vi "vr-main-window.vi"(10 "Robot Num":enum16{"Rob-One", "Rob-Two"}(ring), 11 "EventIn":refnum<class "NISAST Event.lvclass">) -> ()   [LabVIEW 2013]
uses:
  <resource>/importtools/Common/Event/NISAST Event.lvclass
  vr-states.ctl
  <vilib>/picture/3D Picture Control/NI_3D Picture Control.lvlib
panel:
  in  "StopFour":bool
  in  "ClockWise":bool
  in  "AntiClockWise":bool
  in  "Up":bool
  in  "Down":bool
  out "Event Message":string
  out "StopVRWindow?":bool
  in  "Stop":bool
  # "这个名字千万不能改"
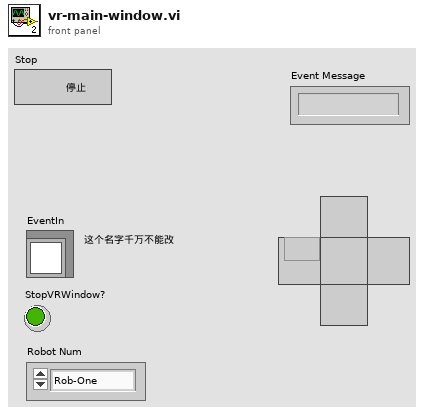
[diagram p1: front panel]
types:
  T1 = typedef "vr-states.ctl" = enum16{"init", "wait", "stopVR", "Ro-Up", "Ro-Down", "Ro-Clockwise", "Ro-AntiClock", "Ro-Stop"}
  T2 = enum16{"Open", "Minimized", "Maximized", "Hidden"}
  T3 = cluster{"zuoqian1":refnum<vi>, "zuoqian2":refnum<vi>, "zuoqian3":refnum<vi>}
  T4 = cluster{"zuohou1":refnum<vi>, "zuohou2":refnum<vi>, "zuohou3":refnum<vi>}
  T5 = cluster{"youqian1":refnum<vi>, "youqian2":refnum<vi>, "youqian3":refnum<vi>}
  T6 = cluster{"youhou1":refnum<vi>, "youhou2":refnum<vi>, "youhou3":refnum<vi>}
  T7 = enum16{"None", "Spherical", "Flying", "Oriented"}
  T8 = typedef "NISAST Event.lvclass/Event Registeration Refnum.ctl" = refnum<event-registration>
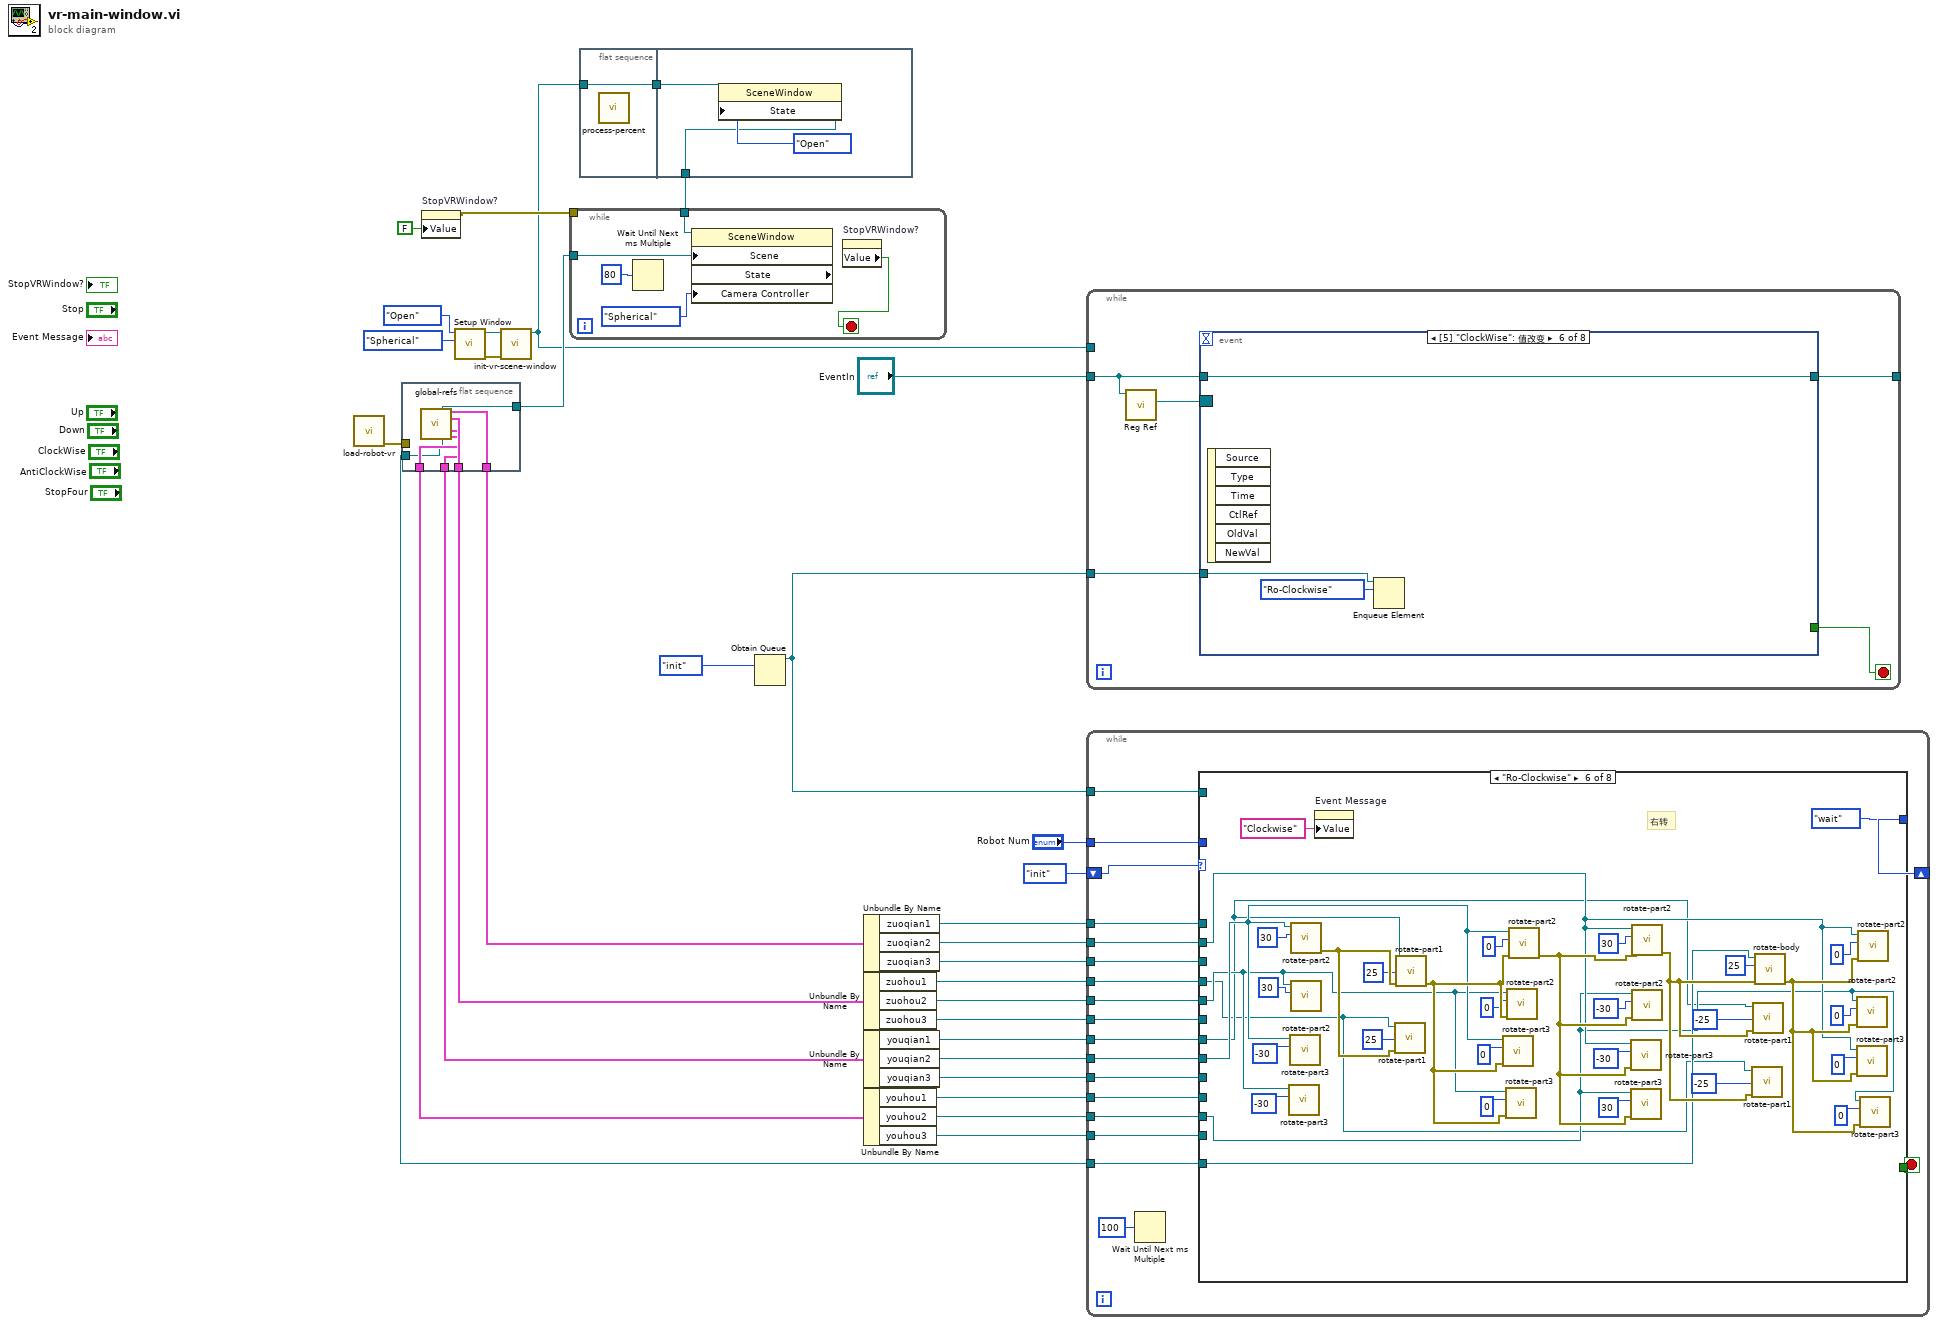
[diagram p0: block diagram]
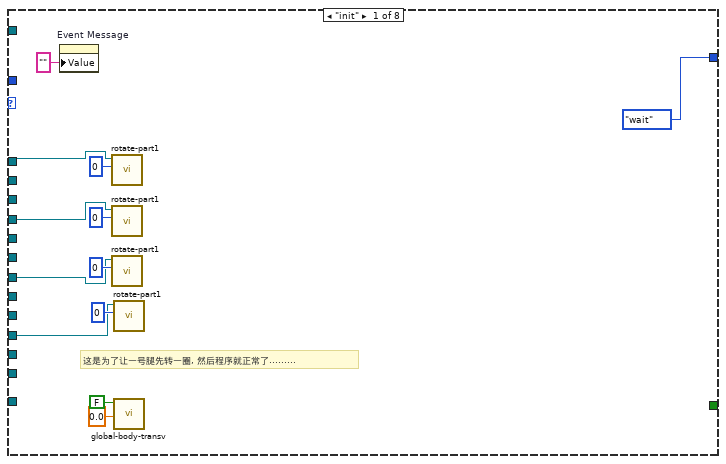
[diagram p2: hidden frame]
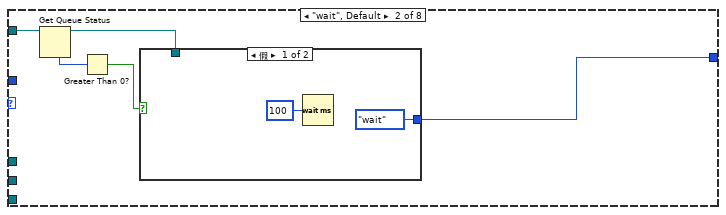
[diagram p3: hidden frame]
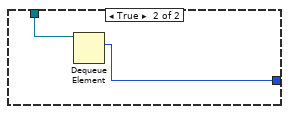
[diagram p4: hidden frame]
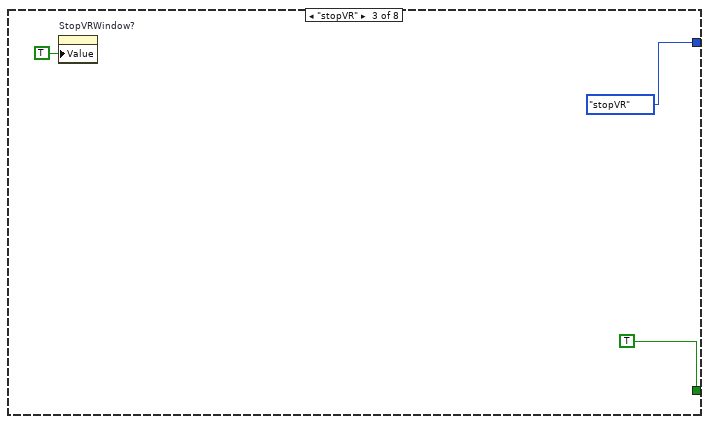
[diagram p5: hidden frame]
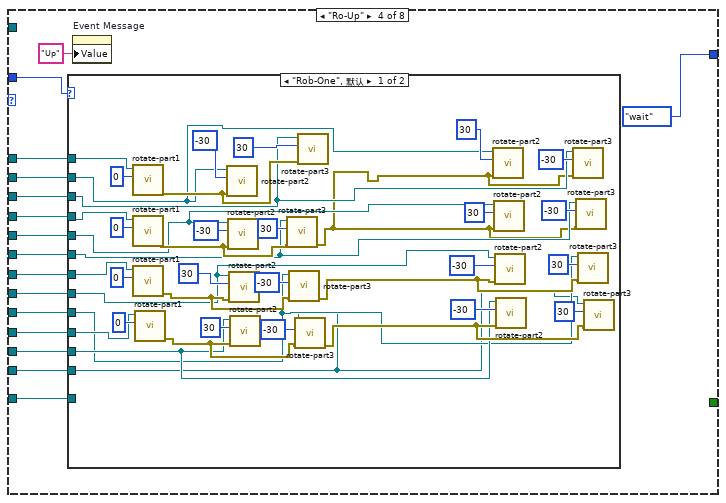
[diagram p6: hidden frame]
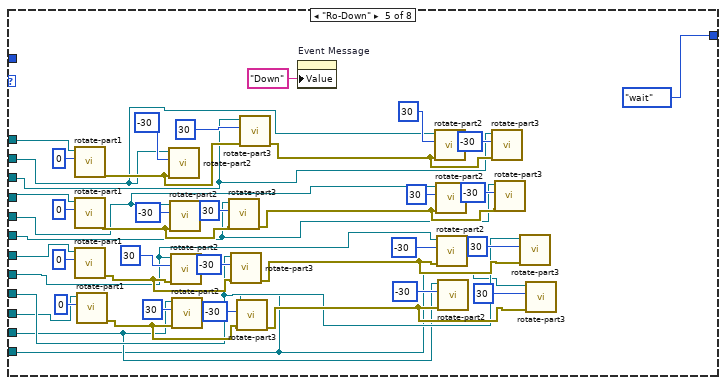
[diagram p8: hidden frame]
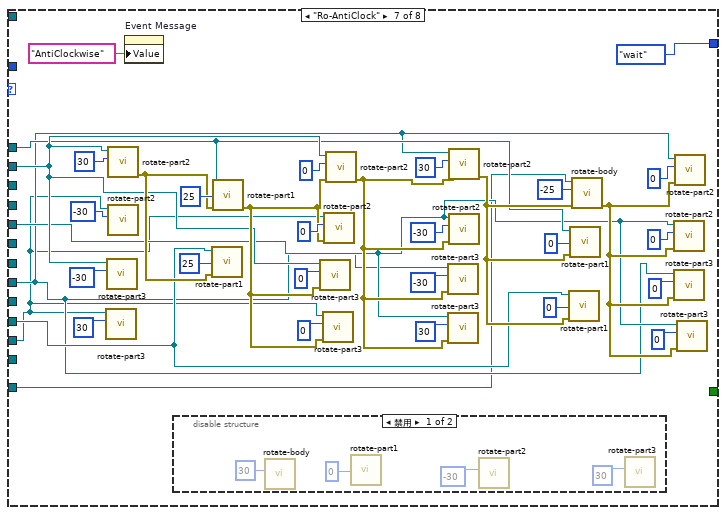
[diagram p9: hidden frame]
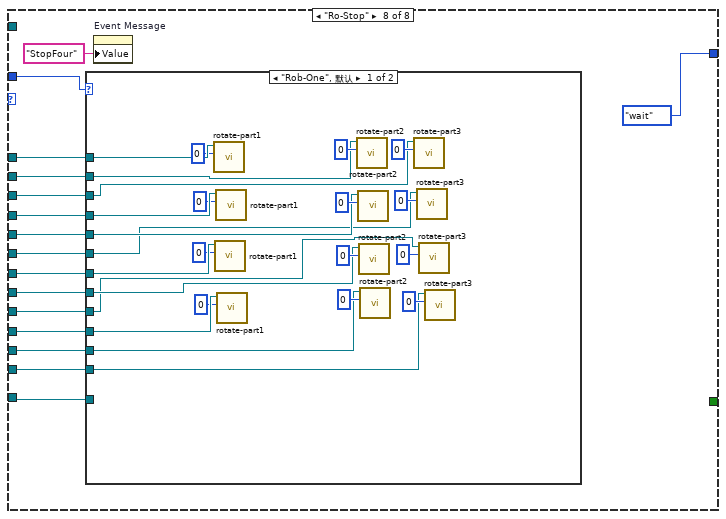
[diagram p11: hidden frame]
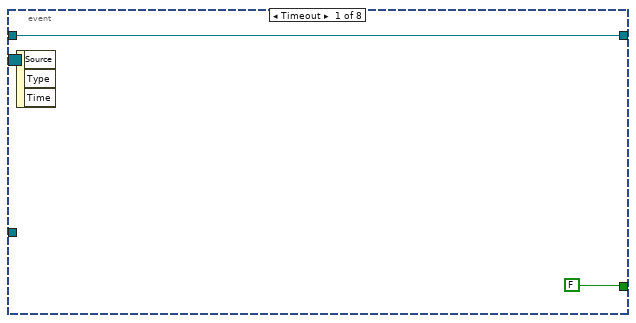
[diagram p13: hidden frame]
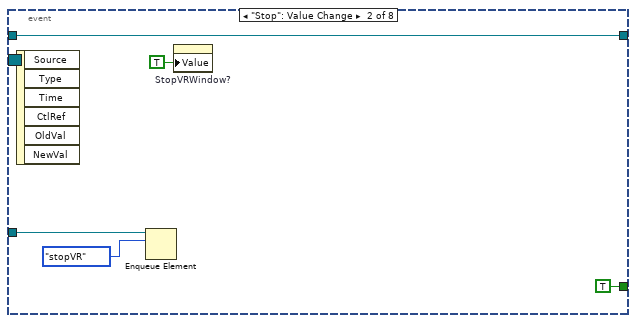
[diagram p14: hidden frame]
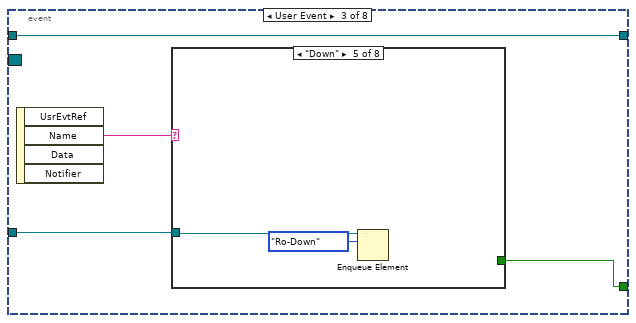
[diagram p15: hidden frame]
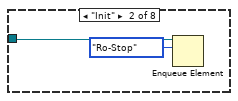
[diagram p17: hidden frame]
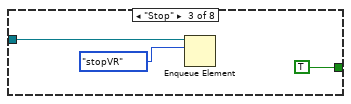
[diagram p18: hidden frame]
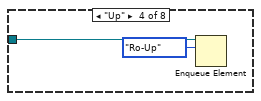
[diagram p19: hidden frame]
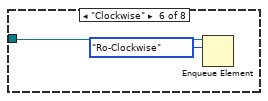
[diagram p20: hidden frame]
diagram:
  n1 = call "load-robot-vr.vi"() -> ("错误输出"=w29:errorcluster)  [unwired: 11 in]
  n2 = flat-sequence {
    tunnel: [w39] -> w27
    tunnel: w29 -> [_]
    tunnel: [w38] -> w28
    tunnel: [w37] -> w21
    tunnel: [w36] -> w20
    tunnel: [w35] -> w19
    tunnel: [w34] -> w6
    frame #0 {
      n3 = call "global-refs.vi"() -> ("RobotRef"=w39:refnum<vi>, "ZuoQianRef"=w38:T3, "ZuoHouRef"=w37:T4, "YouQianRef"=w36:T5, "BodyRef"=w34:refnum<vi>, "YouHouRef"=w35:T6)  [unwired: 10 in]
    }
  }
  n4 = property on="StopVRWindow?" class="Bool (严格)"("Value"=FALSE ("StopVRWindow?")) -> (error out=w4:errorcluster)  [unwired: 2 in, 1 out]
  n5 = call <vilib>:"Setup Window.vi"("Camera Controller"=enum16{"None", "Spherical", "Flying"}."Spherical", "Window State"=T2."Open") -> ("error out"=w33:errorcluster, "New Window Refnum"=w32:refnum<vi>)  [unwired: 1 in, 7 out]
  n6 = call "init-vr-scene-window.vi"("错误输入（无错误）"=w33, "SceneWindow输入"=w32) -> ("SceneWindow输出"=w3:refnum<vi>)  [unwired: 8 in, 1 out]
  n7 = while {
    tunnel: w27 -> [w43]
    tunnel: w1 -> [w42]
    tunnel: w4 -> [_]
    stop <- w40 stop-if-true
    n8 = Wait Until Next ms Multiple(millisecond multiple=u32 80 ("毫秒倍数")) -> ()  [unwired: 1 out]
    n9 = property class="SceneWindow" props=["Scene", "State", "Camera Controller"](reference=w42, "Scene"=w43, "Camera Controller"=T7."Spherical" ("视角控制器:类型")) -> ()  [unwired: 1 in, 3 out]
    n10 = property on="StopVRWindow?" class="Bool (严格)"() -> ("Value"=w40:bool)  [unwired: 2 in, 2 out]
  }
  n11 = flat-sequence {
    tunnel: w3 -> [w45]
    tunnel: [w45] -> w2
    tunnel: w2 -> [w47]
    tunnel: [w46] -> w1
    frame #0 {
      n12 = call "process-percent.vi"() -> ()  [unwired: 12 in]
    }
    frame #1 {
      n13 = property class="SceneWindow"(reference=w47, "State"=T2."Open" ("窗口状态")) -> (reference out=w46:refnum<vi>)  [unwired: 1 in, 1 out]
    }
  }
  n14 = Obtain Queue(element data type=vr-states."init" ("States")) -> (queue out=w25:refnum<queue>)  [unwired: 4 in, 2 out]
  n15 = Unbundle By Name(w28) -> ("zuoqian1"=w18:refnum<vi>, "zuoqian2"=w17:refnum<vi>, "zuoqian3"=w16:refnum<vi>)
  n16 = Unbundle By Name(w21) -> ("zuohou1"=w15:refnum<vi>, "zuohou2"=w14:refnum<vi>, "zuohou3"=w13:refnum<vi>)
  n17 = Unbundle By Name(w20) -> ("youqian1"=w12:refnum<vi>, "youqian2"=w11:refnum<vi>, "youqian3"=w10:refnum<vi>)
  n18 = Unbundle By Name(w19) -> ("youhou1"=w9:refnum<vi>, "youhou2"=w8:refnum<vi>, "youhou3"=w7:refnum<vi>)
  n19 = while {
    tunnel: w3 -> [_]
    tunnel: w25 -> [w53]
    tunnel: "EventIn" -> [w51]
    tunnel: [w49] -> _
    stop <- w52 stop-if-true
    n20 = call-dynamic "Reg Ref.vi"("Event in"=w51) -> ("Event Registration Refnum"=w50:T8)  [unwired: 8 in, 2 out]
    n21 = event shown="[5] \"ClockWise\": 值改变" {
      selector: w50 -> [_ _ _ _ _ _ _ _]
      dyn-events: _ -> [_ _ _ _ _ _ _ _]
      timeout: _ -> [_ _ _ _ _ _ _ _]
      tunnel: w53 -> [_ w59 w63 w81 w84 w87 w90 w93]
      tunnel: [FALSE TRUE w62 _ _ _ _ _] -> w52
      tunnel: w51 -> [w54 w56 w61 w80 w83 w86 w89 w92]
      tunnel: [w54 w56 w61 w80 w83 w86 w89 w92] -> w49
      event Timeout {
        n22 = event-data() -> ()  [unwired: 1 in, 3 out]
      }
      event "Stop": Value Change {
        n23 = event-data() -> ()  [unwired: 1 in, 6 out]
        n24 = Enqueue Element(queue=w59, element=vr-states."stopVR" ("元素")) -> ()  [unwired: 2 in, 3 out]
        n25 = property on="StopVRWindow?" class="Bool (严格)"("Value"=TRUE ("StopVRWindow?")) -> ()  [unwired: 2 in, 2 out]
      }
      event User Event {
        n26 = event-data() -> ("Name"=w64:string)  [unwired: 1 in, 3 out]
        n27 = case shown="\"Down\"" w64 {
          tunnel: w63 -> [_ w66 w68 w70 w72 w74 w76 w78]
          tunnel: [_ _ TRUE _ _ _ _ _] -> w62
          frame "none", Default {
          }
          frame "Init" {
            n28 = Enqueue Element(queue=w66, element=vr-states."Ro-Stop" ("元素")) -> ()  [unwired: 2 in, 3 out]
          }
          frame "Stop" {
            n29 = Enqueue Element(queue=w68, element=vr-states."stopVR" ("元素")) -> ()  [unwired: 2 in, 3 out]
          }
          frame "Up" {
            n30 = Enqueue Element(queue=w70, element=vr-states."Ro-Up" ("元素")) -> ()  [unwired: 2 in, 3 out]
          }
          frame "Down" {
            n31 = Enqueue Element(queue=w72, element=vr-states."Ro-Down" ("元素")) -> ()  [unwired: 2 in, 3 out]
          }
          frame "Clockwise" {
            n32 = Enqueue Element(queue=w74, element=vr-states."Ro-Clockwise" ("元素")) -> ()  [unwired: 2 in, 3 out]
          }
          frame "AntiClockwise" {
            n33 = Enqueue Element(queue=w76, element=vr-states."Ro-AntiClock" ("元素")) -> ()  [unwired: 2 in, 3 out]
          }
          frame "StopFour" {
            n34 = Enqueue Element(queue=w78, element=vr-states."Ro-Stop" ("元素")) -> ()  [unwired: 2 in, 3 out]
          }
        }
      }
      event "Up": Value Change {
        n35 = event-data() -> ()  [unwired: 1 in, 6 out]
        n36 = Enqueue Element(queue=w81, element=vr-states."Ro-Up" ("元素")) -> ()  [unwired: 2 in, 3 out]
      }
      event "Down": Value Change {
        n37 = event-data() -> ()  [unwired: 1 in, 6 out]
        n38 = Enqueue Element(queue=w84, element=vr-states."Ro-Down" ("元素")) -> ()  [unwired: 2 in, 3 out]
      }
      event "ClockWise": Value Change {
        n39 = event-data() -> ()  [unwired: 1 in, 6 out]
        n40 = Enqueue Element(queue=w87, element=vr-states."Ro-Clockwise" ("元素")) -> ()  [unwired: 2 in, 3 out]
      }
      event "AntiClockWise": Value Change {
        n41 = event-data() -> ()  [unwired: 1 in, 6 out]
        n42 = Enqueue Element(queue=w90, element=vr-states."Ro-AntiClock" ("元素")) -> ()  [unwired: 2 in, 3 out]
      }
      event "StopFour": Value Change {
        n43 = event-data() -> ()  [unwired: 1 in, 6 out]
        n44 = Enqueue Element(queue=w93, element=vr-states."Ro-Stop" ("元素")) -> ()  [unwired: 2 in, 3 out]
      }
    }
  }
  n45 = while {
    tunnel: w25 -> [w112]
    shift-right: [w111] -> _
    shift-left: vr-states."init" ("States") -> [w110]
    tunnel: "Robot Num" -> [w109]
    tunnel: w18 -> [w108]
    tunnel: w17 -> [w107]
    tunnel: w16 -> [w106]
    tunnel: w15 -> [w105]
    tunnel: w14 -> [w104]
    tunnel: w13 -> [w103]
    tunnel: w12 -> [w102]
    tunnel: w11 -> [w101]
    tunnel: w10 -> [w100]
    tunnel: w9 -> [w99]
    tunnel: w8 -> [w98]
    tunnel: w7 -> [w97]
    tunnel: w6 -> [w95]
    stop <- w113 stop-if-true
    n46 = Wait Until Next ms Multiple(millisecond multiple=u32 100 ("毫秒倍数")) -> ()  [unwired: 1 out]
    n47 = case shown="\"Ro-Clockwise\"" w110 {
      tunnel: [_ _ TRUE _ _ _ _ _] -> w113
      tunnel: w112 -> [_ w130 _ _ _ _ _ _]
      tunnel: [vr-states."wait" ("States") w126 vr-states."stopVR" ("States") vr-states."wait" ("States") vr-states."wait" ("States") vr-states."wait" ("States") vr-states."wait" ("States") vr-states."wait" ("States")] -> w111
      tunnel: w109 -> [_ _ _ w148 _ _ _ w322]
      tunnel: w108 -> [w119 _ _ w151 w204 _ w275 w321]
      tunnel: w107 -> [_ _ _ w150 w203 w259 w276 w320]
      tunnel: w106 -> [_ _ _ w149 w202 _ _ w319]
      tunnel: w105 -> [w118 _ _ w147 w201 w256 _ w318]
      tunnel: w104 -> [_ _ _ w146 w200 w261 w274 w317]
      tunnel: w103 -> [_ _ _ w145 w199 _ _ w316]
      tunnel: w102 -> [w117 _ _ w144 w198 w257 _ w315]
      tunnel: w101 -> [_ _ _ w143 w197 w262 w272 w314]
      tunnel: w100 -> [_ _ _ w142 w196 _ _ w313]
      tunnel: w99 -> [w116 _ _ w141 w195 _ w273 w312]
      tunnel: w98 -> [_ _ _ w140 w194 w258 w271 w311]
      tunnel: w97 -> [_ _ _ w139 w193 _ _ w310]
      tunnel: w95 -> [_ _ _ w138 _ w260 w270 w309]
      frame "init" {
        # "这是为了让一号腿先转一圈, 然后程序就正常了........."
        n48 = property on="Event Message" class="Str"("Value"="" ("Event Message")) -> ()  [unwired: 2 in, 2 out]
        n49 = call "rotate-part1.vi"("Angle"=0, "SceneObject输入"=w119) -> ()  [unwired: 8 in, 2 out]
        n50 = call "rotate-part1.vi"("Angle"=0, "SceneObject输入"=w118) -> ()  [unwired: 8 in, 2 out]
        n51 = call "rotate-part1.vi"("Angle"=0, "SceneObject输入"=w117) -> ()  [unwired: 8 in, 2 out]
        n52 = call "rotate-part1.vi"("Angle"=0, "SceneObject输入"=w116) -> ()  [unwired: 8 in, 2 out]
        n53 = call "global-body-transv.vi"("rad"=0.0, "Read?"=FALSE) -> ()  [unwired: 8 in, 2 out]
      }
      frame "wait", Default {
        n54 = Get Queue Status(queue=w130) -> (queue out=w127:refnum<queue>, # elements in queue=w129:i32)  [unwired: 2 in, 6 out]
        n55 = Greater Than 0?(x=w129) -> (x > 0?=w128:bool)
        n56 = case shown="假" w128 {
          tunnel: w127 -> [_ w134]
          tunnel: [vr-states."wait" ("States") w133] -> w126
          frame False {
            n57 = Wait (ms)(milliseconds to wait=u32 100 ("等待时间（毫秒）")) -> ()  [unwired: 1 out]
          }
          frame True {
            n58 = Dequeue Element(queue=w134) -> (element=w133:T1)  [unwired: 2 in, 3 out]
          }
        }
      }
      frame "stopVR" {
        n59 = property on="StopVRWindow?" class="Bool (严格)"("Value"=TRUE ("StopVRWindow?")) -> ()  [unwired: 2 in, 2 out]
      }
      frame "Ro-Up" {
        n60 = case shown="\"Rob-One\", 默认" w148 {
          tunnel: w151 -> [w188 _]
          tunnel: w150 -> [w162 _]
          tunnel: w149 -> [w159 _]
          tunnel: w147 -> [w187 _]
          tunnel: w146 -> [w161 _]
          tunnel: w145 -> [w158 _]
          tunnel: w144 -> [w186 _]
          tunnel: w143 -> [w157 _]
          tunnel: w142 -> [w156 _]
          tunnel: w141 -> [w185 _]
          tunnel: w140 -> [w160 _]
          tunnel: w139 -> [w155 _]
          tunnel: w138 -> [_ _]
          frame "Rob-One", Default {
            n61 = call "rotate-part1.vi"("Angle"=0, "SceneObject输入"=w188) -> ("Error Out"=w180:errorcluster)  [unwired: 8 in, 1 out]
            n62 = call "rotate-part1.vi"("Angle"=0, "SceneObject输入"=w187) -> ("Error Out"=w179:errorcluster)  [unwired: 8 in, 1 out]
            n63 = call "rotate-part1.vi"("Angle"=0, "SceneObject输入"=w186) -> ("Error Out"=w178:errorcluster)  [unwired: 8 in, 1 out]
            n64 = call "rotate-part1.vi"("Angle"=0, "SceneObject输入"=w185) -> ("Error Out"=w177:errorcluster)  [unwired: 8 in, 1 out]
            n65 = call "rotate-part2.vi"("Error In"=w180, "Angle"=-30, "SceneObject输入"=w162) -> ()  [unwired: 7 in, 2 out]
            n66 = call "rotate-part2.vi"("Error In"=w179, "Angle"=-30, "SceneObject输入"=w161) -> ()  [unwired: 7 in, 2 out]
            n67 = call "rotate-part2.vi"("Error In"=w178, "Angle"=30, "SceneObject输入"=w157) -> ()  [unwired: 7 in, 2 out]
            n68 = call "rotate-part2.vi"("Error In"=w177, "Angle"=30, "SceneObject输入"=w160) -> ()  [unwired: 7 in, 2 out]
            n69 = call "rotate-part3.vi"("Error In"=w179, "Angle"=30, "SceneObject输入"=w158) -> ("Error Out"=w154:errorcluster)  [unwired: 7 in, 1 out]
            n70 = call "rotate-part3.vi"("Error In"=w178, "Angle"=-30, "SceneObject输入"=w156) -> ("Error Out"=w164:errorcluster)  [unwired: 7 in, 1 out]
            n71 = call "rotate-part3.vi"("Error In"=w177, "Angle"=-30, "SceneObject输入"=w155) -> ("Error Out"=w163:errorcluster)  [unwired: 7 in, 1 out]
            n72 = call "rotate-part3.vi"("Error In"=w180, "Angle"=30, "SceneObject输入"=w159) -> ()  [unwired: 7 in, 2 out]
            n73 = call "rotate-part2.vi"("Error In"=w154, "Angle"=30, "SceneObject输入"=w162) -> ()  [unwired: 7 in, 2 out]
            n74 = call "rotate-part2.vi"("Error In"=w154, "Angle"=30, "SceneObject输入"=w161) -> ()  [unwired: 7 in, 2 out]
            n75 = call "rotate-part2.vi"("Error In"=w164, "Angle"=-30, "SceneObject输入"=w157) -> ()  [unwired: 7 in, 2 out]
            n76 = call "rotate-part2.vi"("Error In"=w163, "Angle"=-30, "SceneObject输入"=w160) -> ()  [unwired: 7 in, 2 out]
            n77 = call "rotate-part3.vi"("Error In"=w154, "Angle"=-30, "SceneObject输入"=w159) -> ()  [unwired: 7 in, 2 out]
            n78 = call "rotate-part3.vi"("Error In"=w154, "Angle"=-30, "SceneObject输入"=w158) -> ()  [unwired: 7 in, 2 out]
            n79 = call "rotate-part3.vi"("Error In"=w164, "Angle"=30, "SceneObject输入"=w156) -> ()  [unwired: 7 in, 2 out]
            n80 = call "rotate-part3.vi"("Error In"=w163, "Angle"=30, "SceneObject输入"=w155) -> ()  [unwired: 7 in, 2 out]
          }
          frame "Rob-Two" {
          }
        }
        n81 = property on="Event Message" class="Str"("Value"="Up" ("Event Message")) -> ()  [unwired: 2 in, 2 out]
      }
      frame "Ro-Down" {
        n82 = call "rotate-part1.vi"("Angle"=0, "SceneObject输入"=w204) -> ("Error Out"=w224:errorcluster)  [unwired: 8 in, 1 out]
        n83 = call "rotate-part1.vi"("Angle"=0, "SceneObject输入"=w201) -> ("Error Out"=w223:errorcluster)  [unwired: 8 in, 1 out]
        n84 = call "rotate-part1.vi"("Angle"=0, "SceneObject输入"=w198) -> ("Error Out"=w222:errorcluster)  [unwired: 8 in, 1 out]
        n85 = call "rotate-part1.vi"("Angle"=0, "SceneObject输入"=w195) -> ("Error Out"=w221:errorcluster)  [unwired: 8 in, 1 out]
        n86 = call "rotate-part2.vi"("Error In"=w224, "Angle"=-30, "SceneObject输入"=w203) -> ()  [unwired: 7 in, 2 out]
        n87 = call "rotate-part2.vi"("Error In"=w223, "Angle"=-30, "SceneObject输入"=w200) -> ()  [unwired: 7 in, 2 out]
        n88 = call "rotate-part2.vi"("Error In"=w222, "Angle"=30, "SceneObject输入"=w197) -> ()  [unwired: 7 in, 2 out]
        n89 = call "rotate-part2.vi"("Error In"=w221, "Angle"=30, "SceneObject输入"=w194) -> ()  [unwired: 7 in, 2 out]
        n90 = call "rotate-part3.vi"("Error In"=w223, "Angle"=30, "SceneObject输入"=w199) -> ("Error Out"=w207:errorcluster)  [unwired: 7 in, 1 out]
        n91 = call "rotate-part3.vi"("Error In"=w222, "Angle"=-30, "SceneObject输入"=w196) -> ("Error Out"=w206:errorcluster)  [unwired: 7 in, 1 out]
        n92 = call "rotate-part3.vi"("Error In"=w221, "Angle"=-30, "SceneObject输入"=w193) -> ("Error Out"=w205:errorcluster)  [unwired: 7 in, 1 out]
        n93 = call "rotate-part3.vi"("Error In"=w224, "Angle"=30, "SceneObject输入"=w202) -> ("Error Out"=w208:errorcluster)  [unwired: 7 in, 1 out]
        n94 = property on="Event Message" class="Str"("Value"="Down" ("Event Message")) -> ()  [unwired: 2 in, 2 out]
        n95 = call "rotate-part2.vi"("Error In"=w208, "Angle"=30, "SceneObject输入"=w203) -> ()  [unwired: 7 in, 2 out]
        n96 = call "rotate-part2.vi"("Error In"=w207, "Angle"=30, "SceneObject输入"=w200) -> ()  [unwired: 7 in, 2 out]
        n97 = call "rotate-part2.vi"("Error In"=w206, "Angle"=-30, "SceneObject输入"=w197) -> ()  [unwired: 7 in, 2 out]
        n98 = call "rotate-part2.vi"("Error In"=w205, "Angle"=-30, "SceneObject输入"=w194) -> ()  [unwired: 7 in, 2 out]
        n99 = call "rotate-part3.vi"("Error In"=w208, "Angle"=-30, "SceneObject输入"=w202) -> ()  [unwired: 7 in, 2 out]
        n100 = call "rotate-part3.vi"("Error In"=w207, "Angle"=-30, "SceneObject输入"=w199) -> ()  [unwired: 7 in, 2 out]
        n101 = call "rotate-part3.vi"("Error In"=w206, "Angle"=30, "SceneObject输入"=w196) -> ()  [unwired: 7 in, 2 out]
        n102 = call "rotate-part3.vi"("Error In"=w205, "Angle"=30, "SceneObject输入"=w193) -> ()  [unwired: 7 in, 2 out]
      }
      frame "Ro-Clockwise" {
        # "右转"
        n103 = call "rotate-part3.vi"("Angle"=-30, "SceneObject输入"=w261) -> ()  [unwired: 8 in, 2 out]
        n104 = call "rotate-part3.vi"("Angle"=-30, "SceneObject输入"=w262) -> ()  [unwired: 8 in, 2 out]
        n105 = call "rotate-part2.vi"("Angle"=30, "SceneObject输入"=w262) -> ("Error Out"=w267:errorcluster)  [unwired: 8 in, 1 out]
        n106 = call "rotate-part2.vi"("Angle"=30, "SceneObject输入"=w261) -> ()  [unwired: 8 in, 2 out]
        n107 = property on="Event Message" class="Str"("Value"="Clockwise" ("Event Message")) -> ()  [unwired: 2 in, 2 out]
        n108 = call "rotate-part1.vi"("Error In"=w267, "Angle"=25, "SceneObject输入"=w256) -> ()  [unwired: 7 in, 2 out]
        n109 = call "rotate-part1.vi"("Error In"=w267, "Angle"=25, "SceneObject输入"=w257) -> ("Error Out"=w265:errorcluster)  [unwired: 7 in, 1 out]
        n110 = call "rotate-part3.vi"("Error In"=w265, "Angle"=0, "SceneObject输入"=w262) -> ()  [unwired: 7 in, 2 out]
        n111 = call "rotate-part3.vi"("Error In"=w265, "Angle"=0, "SceneObject输入"=w261) -> ()  [unwired: 7 in, 2 out]
        n112 = call "rotate-part2.vi"("Error In"=w265, "Angle"=0, "SceneObject输入"=w261) -> ()  [unwired: 7 in, 2 out]
        n113 = call "rotate-part2.vi"("Error In"=w265, "Angle"=0, "SceneObject输入"=w262) -> ("Error Out"=w266:errorcluster)  [unwired: 7 in, 1 out]
        n114 = call "rotate-part3.vi"("Error In"=w266, "Angle"=-30, "SceneObject输入"=w259) -> ()  [unwired: 7 in, 2 out]
        n115 = call "rotate-part3.vi"("Error In"=w266, "Angle"=30, "SceneObject输入"=w258) -> ()  [unwired: 7 in, 2 out]
        n116 = call "rotate-part2.vi"("Error In"=w266, "Angle"=30, "SceneObject输入"=w259) -> ("Error Out"=w264:errorcluster)  [unwired: 7 in, 1 out]
        n117 = call "rotate-part2.vi"("Error In"=w266, "Angle"=-30, "SceneObject输入"=w258) -> ()  [unwired: 7 in, 2 out]
        n118 = call "rotate-part1.vi"("Error In"=w264, "Angle"=-25, "SceneObject输入"=w256) -> ()  [unwired: 7 in, 2 out]
        n119 = call "rotate-part1.vi"("Error In"=w264, "Angle"=-25, "SceneObject输入"=w257) -> ()  [unwired: 7 in, 2 out]
        n120 = call "rotate-body.vi"("Error In"=w264, "Angle"=25, "SceneObject输入"=w260) -> ("Error Out"=w263:errorcluster)  [unwired: 7 in, 1 out]
        n121 = call "rotate-part2.vi"("Error In"=w263, "Angle"=0, "SceneObject输入"=w258) -> ()  [unwired: 7 in, 2 out]
        n122 = call "rotate-part3.vi"("Error In"=w263, "Angle"=0, "SceneObject输入"=w259) -> ()  [unwired: 7 in, 2 out]
        n123 = call "rotate-part2.vi"("Error In"=w263, "Angle"=0, "SceneObject输入"=w259) -> ()  [unwired: 7 in, 2 out]
        n124 = call "rotate-part3.vi"("Error In"=w263, "Angle"=0, "SceneObject输入"=w258) -> ()  [unwired: 7 in, 2 out]
      }
      frame "Ro-AntiClock" {
        n125 = call "rotate-part3.vi"("Angle"=30, "SceneObject输入"=w271) -> ()  [unwired: 8 in, 2 out]
        n126 = call "rotate-part3.vi"("Angle"=-30, "SceneObject输入"=w276) -> ()  [unwired: 8 in, 2 out]
        n127 = call "rotate-part2.vi"("Angle"=30, "SceneObject输入"=w276) -> ("Error Out"=w282:errorcluster)  [unwired: 8 in, 1 out]
        n128 = call "rotate-part2.vi"("Angle"=-30, "SceneObject输入"=w271) -> ()  [unwired: 8 in, 2 out]
        n129 = property on="Event Message" class="Str"("Value"="AntiClockwise" ("Event Message")) -> ()  [unwired: 2 in, 2 out]
        n130 = disable-structure shown="禁用" {
          frame Disabled {
            n131 = call "rotate-body.vi"("Angle"=30) -> ()  [unwired: 9 in, 2 out]
            n132 = call "rotate-part1.vi"("Angle"=0) -> ()  [unwired: 9 in, 2 out]
            n133 = call "rotate-part2.vi"("Angle"=-30) -> ()  [unwired: 9 in, 2 out]
            n134 = call "rotate-part3.vi"("Angle"=30) -> ()  [unwired: 9 in, 2 out]
          }
          frame Enabled {
          }
        }
        n135 = call "rotate-part1.vi"("Error In"=w282, "Angle"=25, "SceneObject输入"=w273) -> ()  [unwired: 7 in, 2 out]
        n136 = call "rotate-part1.vi"("Error In"=w282, "Angle"=25, "SceneObject输入"=w275) -> ("Error Out"=w280:errorcluster)  [unwired: 7 in, 1 out]
        n137 = call "rotate-part3.vi"("Error In"=w280, "Angle"=0, "SceneObject输入"=w276) -> ()  [unwired: 7 in, 2 out]
        n138 = call "rotate-part3.vi"("Error In"=w280, "Angle"=0, "SceneObject输入"=w271) -> ()  [unwired: 7 in, 2 out]
        n139 = call "rotate-part2.vi"("Error In"=w280, "Angle"=0, "SceneObject输入"=w271) -> ()  [unwired: 7 in, 2 out]
        n140 = call "rotate-part2.vi"("Error In"=w280, "Angle"=0, "SceneObject输入"=w276) -> ("Error Out"=w281:errorcluster)  [unwired: 7 in, 1 out]
        n141 = call "rotate-part3.vi"("Error In"=w281, "Angle"=-30, "SceneObject输入"=w272) -> ()  [unwired: 7 in, 2 out]
        n142 = call "rotate-part3.vi"("Error In"=w281, "Angle"=30, "SceneObject输入"=w274) -> ()  [unwired: 7 in, 2 out]
        n143 = call "rotate-part2.vi"("Error In"=w281, "Angle"=30, "SceneObject输入"=w272) -> ("Error Out"=w278:errorcluster)  [unwired: 7 in, 1 out]
        n144 = call "rotate-part2.vi"("Error In"=w281, "Angle"=-30, "SceneObject输入"=w274) -> ()  [unwired: 7 in, 2 out]
        n145 = call "rotate-part1.vi"("Error In"=w278, "Angle"=0, "SceneObject输入"=w273) -> ()  [unwired: 7 in, 2 out]
        n146 = call "rotate-part1.vi"("Error In"=w278, "Angle"=0, "SceneObject输入"=w275) -> ()  [unwired: 7 in, 2 out]
        n147 = call "rotate-body.vi"("Error In"=w278, "Angle"=-25, "SceneObject输入"=w270) -> ("Error Out"=w277:errorcluster)  [unwired: 7 in, 1 out]
        n148 = call "rotate-part2.vi"("Error In"=w277, "Angle"=0, "SceneObject输入"=w274) -> ()  [unwired: 7 in, 2 out]
        n149 = call "rotate-part3.vi"("Error In"=w277, "Angle"=0, "SceneObject输入"=w272) -> ()  [unwired: 7 in, 2 out]
        n150 = call "rotate-part2.vi"("Error In"=w277, "Angle"=0, "SceneObject输入"=w272) -> ()  [unwired: 7 in, 2 out]
        n151 = call "rotate-part3.vi"("Error In"=w277, "Angle"=0, "SceneObject输入"=w274) -> ()  [unwired: 7 in, 2 out]
      }
      frame "Ro-Stop" {
        n152 = case shown="\"Rob-One\", 默认" w322 {
          tunnel: w321 -> [w348 _]
          tunnel: w320 -> [w332 _]
          tunnel: w319 -> [w328 _]
          tunnel: w318 -> [w347 _]
          tunnel: w317 -> [w331 _]
          tunnel: w316 -> [w327 _]
          tunnel: w315 -> [w346 _]
          tunnel: w314 -> [w330 _]
          tunnel: w313 -> [w326 _]
          tunnel: w312 -> [w345 _]
          tunnel: w311 -> [w329 _]
          tunnel: w310 -> [w325 _]
          tunnel: w309 -> [_ _]
          frame "Rob-One", Default {
            n153 = call "rotate-part1.vi"("Angle"=0, "SceneObject输入"=w348) -> ()  [unwired: 8 in, 2 out]
            n154 = call "rotate-part1.vi"("Angle"=0, "SceneObject输入"=w346) -> ()  [unwired: 8 in, 2 out]
            n155 = call "rotate-part1.vi"("Angle"=0, "SceneObject输入"=w347) -> ()  [unwired: 8 in, 2 out]
            n156 = call "rotate-part1.vi"("Angle"=0, "SceneObject输入"=w345) -> ()  [unwired: 8 in, 2 out]
            n157 = call "rotate-part2.vi"("Angle"=0, "SceneObject输入"=w332) -> ()  [unwired: 8 in, 2 out]
            n158 = call "rotate-part2.vi"("Angle"=0, "SceneObject输入"=w331) -> ()  [unwired: 8 in, 2 out]
            n159 = call "rotate-part2.vi"("Angle"=0, "SceneObject输入"=w330) -> ()  [unwired: 8 in, 2 out]
            n160 = call "rotate-part2.vi"("Angle"=0, "SceneObject输入"=w329) -> ()  [unwired: 8 in, 2 out]
            n161 = call "rotate-part3.vi"("Angle"=0, "SceneObject输入"=w328) -> ()  [unwired: 8 in, 2 out]
            n162 = call "rotate-part3.vi"("Angle"=0, "SceneObject输入"=w327) -> ()  [unwired: 8 in, 2 out]
            n163 = call "rotate-part3.vi"("Angle"=0, "SceneObject输入"=w326) -> ()  [unwired: 8 in, 2 out]
            n164 = call "rotate-part3.vi"("Angle"=0, "SceneObject输入"=w325) -> ()  [unwired: 8 in, 2 out]
          }
          frame "Rob-Two" {
          }
        }
        n165 = property on="Event Message" class="Str"("Value"="StopFour" ("Event Message")) -> ()  [unwired: 2 in, 2 out]
      }
    }
  }
